vi "Initialize (FPGA).vi"(8 "error in (no error)":errorcluster, 10 "Sensor ID (0)":i32, 11 "FPGA VI Reference":refnum<k20>) -> (0 "error out":errorcluster, 3 "Parallax PING))) out":refnum<class "Parallax PING))).lvclass">)   [LabVIEW 2013, in "Parallax PING))) FPGA.lvclass"]
doc: "Establishes communication with the sensor. Therefore, call this VI before calling other sensor driver VIs for this sensor. Generally, you need to call the Initialize VI only once at the beginning of an application.\n\n<B>Notes:</B>\nPlease refer to the example project in the FPGA Example folder of this driver for how to configure the FPGA target and use this VI."
uses:
  Parallax PING))) FPGA.lvclass
  Parallax PING))).lvclass
  Parallax PING))) FPGA.lvclass/Parallax PING))) FPGA.ctl
panel:
  # "(c) 2011 National Instruments.  ALL RIGHTS RESERVED."
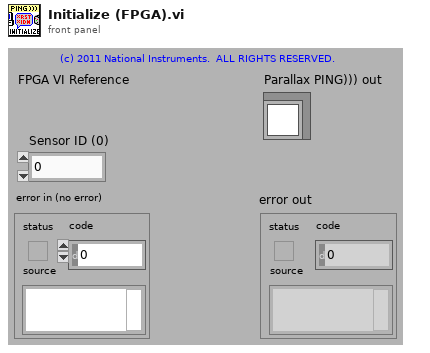
[diagram p1: front panel]
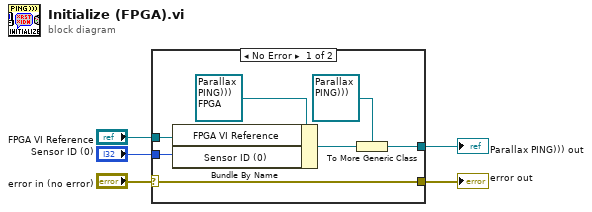
[diagram p0: block diagram]
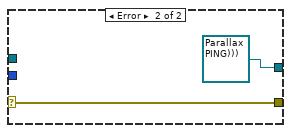
[diagram p2: hidden frame]
diagram:
  n1 = case shown="No Error" "error in (no error)" {
    selector: "error in (no error)" -> [w10 w14]
    tunnel: "FPGA VI Reference" -> [w11 _]
    tunnel: [w10 w14] -> w3
    tunnel: [w7 refnum<class "Parallax PING))).lvclass"> refnum ("Vishay TEMT6000 FPGA in")] -> w2
    tunnel: "Sensor ID (0)" -> [w6 _]
    frame No Error {
      n2 = Bundle By Name(cluster=refnum<class "Parallax PING))) FPGA.lvclass"> refnum ("Vishay TEMT6000 FPGA in"), "FPGA VI Reference"=w11, "Sensor ID (0)"=w6) -> (w9:refnum<class "Parallax PING))) FPGA.lvclass">)
      n3 = To More Generic Class(target class=refnum<class "Parallax PING))).lvclass"> refnum ("Parallax PING))).lvclass"), reference=w9) -> (generic class reference=w7:refnum<class "Parallax PING))).lvclass">)
    }
    frame Error {
    }
  }
  "Parallax PING))) out" <- w2
  "error out" <- w3
